vi "Vision 표지판 인식.vi"() -> ()   [LabVIEW 2016]
uses:
  <vilib>/vision/Classification.llb/IMAQ Classifier Nearest Neighbor options.ctl
  <vilib>/vision/NI_Vision_Development_Module.lvlib
  <vilib>/ptbypt/NI_PtbyPt.lvlib
panel:
  in  "Colors (Green)":u32[](array[colorbox])=[65280]
  in  "경로 설정":enum32{"주차", "유턴", "곡선", "동적"}(tab)
  in  "File Path (Particle Classification 1)":path=path "C:/Users/SeongHyeon/Desktop/[Github]_GPS Team/labview_program/작업중인 모든 Vi, dll파일 모음/전체프로그램/Sub Vi/Sensor/Vision Reference/주차.clf"
  in  "유턴File Path":path=path "C:/Users/SeongHyeon/Desktop/[Github]_GPS Team/labview_program/작업중인 모든 Vi, dll파일 모음/전체프로그램/Sub Vi/Sensor/Vision Reference/유턴2.clf"
  in  "곡선File Path 2":path=path "C:/Users/SeongHyeon/Desktop/[Github]_GPS Team/labview_program/작업중인 모든 Vi, dll파일 모음/전체프로그램/Sub Vi/Sensor/Vision Reference/곡선2.clf"
  in  "동적장애물File Path 4":path=path "C:/Users/SeongHyeon/Desktop/[Github]_GPS Team/labview_program/작업중인 모든 Vi, dll파일 모음/전체프로그램/Sub Vi/Sensor/Vision Reference/동적 장애물 Dark.clf"
  in  "Parameter 설정":enum32{"주차", "유턴", "곡선", "동적"}(tab)
  in  "주차 Paramaters":T2={"Preprocessing Options"={"Method"=-1, "Looking for"=1, "Threshold Range"={"Lower value"=0.0, "Upper value"=0.0}, "Threshold Limits"={"Lower value"=0.0, "Upper value"=0.0}, "Reject Border"=FALSE, "# of Erosions"=0, "Kernel Size"={"Lower value"=0, "Upper value"=0}, "Deviation Factor"=0.0}, "Nearest Neighbor Options"={"Method"=0, "Metric"=0, "k"=0}, "Particle Options"={"Scale Dependant"=FALSE, "Scale Factor"=0.0, "Symmetry Dependant"=FALSE, "Symmetry Factor"=0.0}} {"Preprocessing Options"."Deviation Factor" min=0.0; "Preprocessing Options"."Threshold Limits"."Upper value" format="%.2f"; "Preprocessing Options"."Threshold Limits"."Lower value" format="%.2f"; "Preprocessing Options"."Threshold Range"."Upper value" format="%.2f"; "Preprocessing Options"."Threshold Range"."Lower value" format="%.2f"; "Preprocessing Options"."# of Erosions" min=0; "Preprocessing Options"."Method" items=["Manual Threshold"=-1, "-"=-2, "Auto Threshold: Clustering"=0, "Auto Threshold: Entropy"=1, "Auto Threshold: Metric"=2, "Auto Threshold: Moments"=3, "Auto Threshold: Inter-class Variance"=4, "--"=-3, "Local Threshold: Niblack"=5, "Local Threshold: BG Correction"=6]; "Preprocessing Options"."Looking for" items=["Bright Objects", "Dark Objects"]; "Nearest Neighbor Options"."Method" items=["Nearest Neighbor", "K Nearest Neighbor", "Minimum Mean Distance"]; "Nearest Neighbor Options"."Metric" items=["Maximum", "Sum", "Euclidean"]; "Nearest Neighbor Options"."k" min=3}
  in  "유턴 Paramaters":T2={"Preprocessing Options"={"Method"=-1, "Looking for"=1, "Threshold Range"={"Lower value"=0.0, "Upper value"=0.0}, "Threshold Limits"={"Lower value"=0.0, "Upper value"=0.0}, "Reject Border"=FALSE, "# of Erosions"=0, "Kernel Size"={"Lower value"=0, "Upper value"=0}, "Deviation Factor"=0.0}, "Nearest Neighbor Options"={"Method"=0, "Metric"=0, "k"=0}, "Particle Options"={"Scale Dependant"=FALSE, "Scale Factor"=0.0, "Symmetry Dependant"=FALSE, "Symmetry Factor"=0.0}} {"Preprocessing Options"."Deviation Factor" min=0.0; "Preprocessing Options"."Threshold Limits"."Upper value" format="%.2f"; "Preprocessing Options"."Threshold Limits"."Lower value" format="%.2f"; "Preprocessing Options"."Threshold Range"."Upper value" format="%.2f"; "Preprocessing Options"."Threshold Range"."Lower value" format="%.2f"; "Preprocessing Options"."# of Erosions" min=0; "Preprocessing Options"."Method" items=["Manual Threshold"=-1, "-"=-2, "Auto Threshold: Clustering"=0, "Auto Threshold: Entropy"=1, "Auto Threshold: Metric"=2, "Auto Threshold: Moments"=3, "Auto Threshold: Inter-class Variance"=4, "--"=-3, "Local Threshold: Niblack"=5, "Local Threshold: BG Correction"=6]; "Preprocessing Options"."Looking for" items=["Bright Objects", "Dark Objects"]; "Nearest Neighbor Options"."Method" items=["Nearest Neighbor", "K Nearest Neighbor", "Minimum Mean Distance"]; "Nearest Neighbor Options"."Metric" items=["Maximum", "Sum", "Euclidean"]; "Nearest Neighbor Options"."k" min=3}
  in  "곡선 Paramaters":T2={"Preprocessing Options"={"Method"=-1, "Looking for"=1, "Threshold Range"={"Lower value"=0.0, "Upper value"=0.0}, "Threshold Limits"={"Lower value"=0.0, "Upper value"=0.0}, "Reject Border"=FALSE, "# of Erosions"=0, "Kernel Size"={"Lower value"=0, "Upper value"=0}, "Deviation Factor"=0.0}, "Nearest Neighbor Options"={"Method"=0, "Metric"=0, "k"=0}, "Particle Options"={"Scale Dependant"=FALSE, "Scale Factor"=0.0, "Symmetry Dependant"=FALSE, "Symmetry Factor"=0.0}} {"Preprocessing Options"."Deviation Factor" min=0.0; "Preprocessing Options"."Threshold Limits"."Upper value" format="%.2f"; "Preprocessing Options"."Threshold Limits"."Lower value" format="%.2f"; "Preprocessing Options"."Threshold Range"."Upper value" format="%.2f"; "Preprocessing Options"."Threshold Range"."Lower value" format="%.2f"; "Preprocessing Options"."# of Erosions" min=0; "Preprocessing Options"."Method" items=["Manual Threshold"=-1, "-"=-2, "Auto Threshold: Clustering"=0, "Auto Threshold: Entropy"=1, "Auto Threshold: Metric"=2, "Auto Threshold: Moments"=3, "Auto Threshold: Inter-class Variance"=4, "--"=-3, "Local Threshold: Niblack"=5, "Local Threshold: BG Correction"=6]; "Preprocessing Options"."Looking for" items=["Bright Objects", "Dark Objects"]; "Nearest Neighbor Options"."Method" items=["Nearest Neighbor", "K Nearest Neighbor", "Minimum Mean Distance"]; "Nearest Neighbor Options"."Metric" items=["Maximum", "Sum", "Euclidean"]; "Nearest Neighbor Options"."k" min=3}
  in  "동적 Paramaters":T2={"Preprocessing Options"={"Method"=-1, "Looking for"=1, "Threshold Range"={"Lower value"=0.0, "Upper value"=0.0}, "Threshold Limits"={"Lower value"=0.0, "Upper value"=0.0}, "Reject Border"=FALSE, "# of Erosions"=0, "Kernel Size"={"Lower value"=0, "Upper value"=0}, "Deviation Factor"=0.0}, "Nearest Neighbor Options"={"Method"=0, "Metric"=0, "k"=0}, "Particle Options"={"Scale Dependant"=FALSE, "Scale Factor"=0.0, "Symmetry Dependant"=FALSE, "Symmetry Factor"=0.0}} {"Preprocessing Options"."Deviation Factor" min=0.0; "Preprocessing Options"."Threshold Limits"."Upper value" format="%.2f"; "Preprocessing Options"."Threshold Limits"."Lower value" format="%.2f"; "Preprocessing Options"."Threshold Range"."Upper value" format="%.2f"; "Preprocessing Options"."Threshold Range"."Lower value" format="%.2f"; "Preprocessing Options"."# of Erosions" min=0; "Preprocessing Options"."Method" items=["Manual Threshold"=-1, "-"=-2, "Auto Threshold: Clustering"=0, "Auto Threshold: Entropy"=1, "Auto Threshold: Metric"=2, "Auto Threshold: Moments"=3, "Auto Threshold: Inter-class Variance"=4, "--"=-3, "Local Threshold: Niblack"=5, "Local Threshold: BG Correction"=6]; "Preprocessing Options"."Looking for" items=["Bright Objects", "Dark Objects"]; "Nearest Neighbor Options"."Method" items=["Nearest Neighbor", "K Nearest Neighbor", "Minimum Mean Distance"]; "Nearest Neighbor Options"."Metric" items=["Maximum", "Sum", "Euclidean"]; "Nearest Neighbor Options"."k" min=3}
  out "동적이냐":bool
  out "곡선이냐":bool
  out "횡단보도 거리":dbl[](array[numeric])
  out "유턴이냐":bool
  in  "ROI Descriptor (Particle Classification 1) 2":T3={"Global Rectangle"=[750, 250, 1250, 750], "Contours"=[{"ID"=enum."External", "Type"=3, "Coordinates"=[750, 399, 891, 593]}]} {"Contours"."Type" items=["No Selection", "Point", "Line", "Rectangle", "Oval", "Polygon", "Freehand Region", "Annulus", "Unused2", "Unused3", "Broken Line", "Freehand Line", "Rotated Rectangle"]}
  in  "Stop (F)":bool
  out "Image":T4(plugin-control)
  out "Identification Score":sgl
  out "주차냐":bool
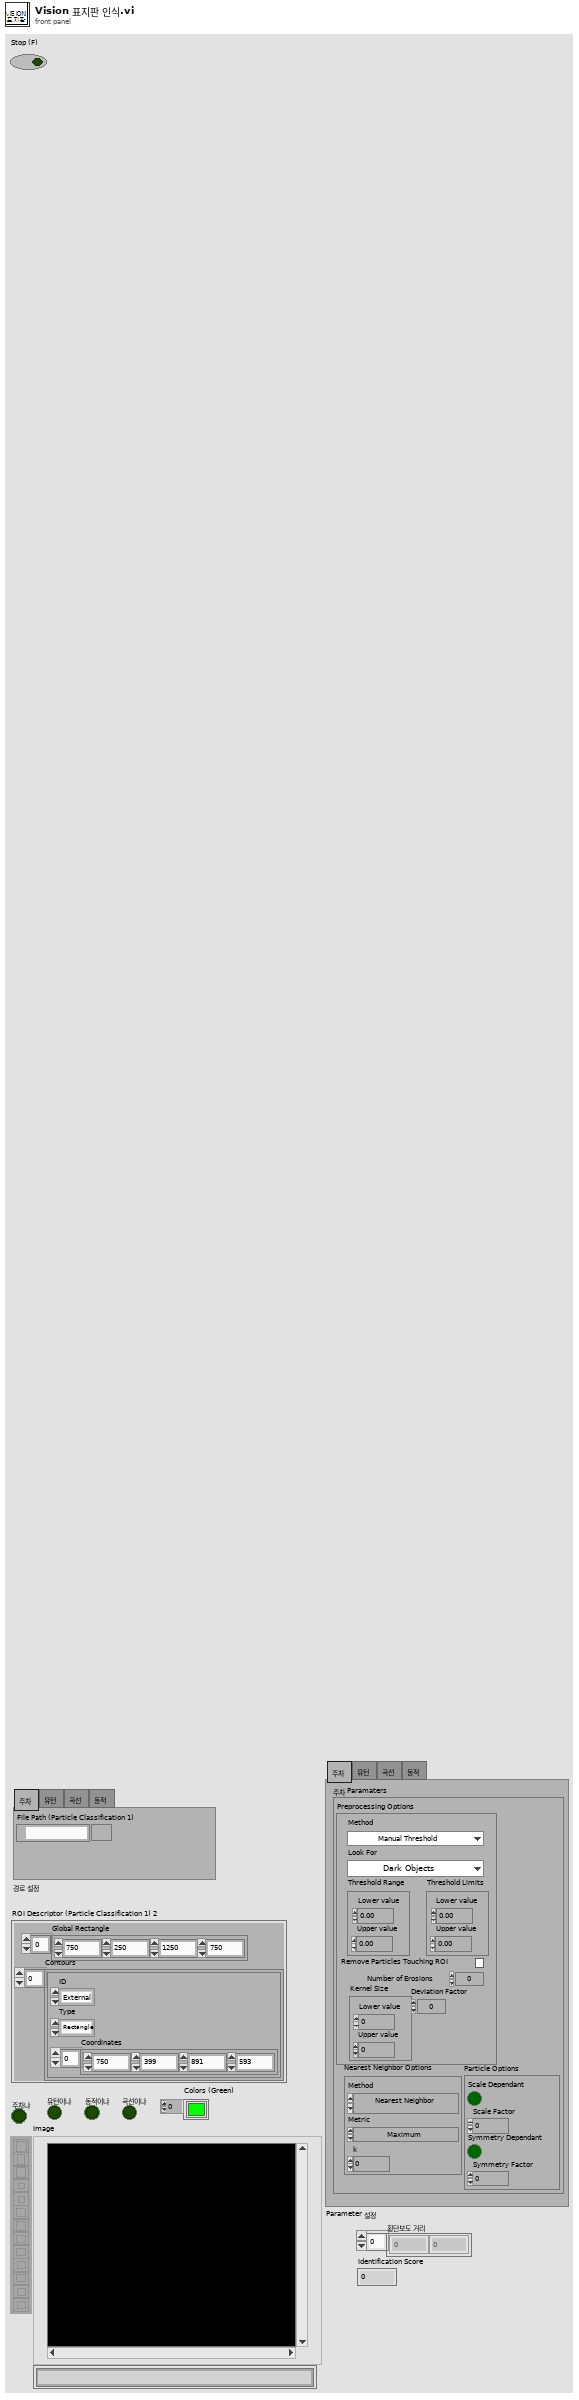
[diagram p1: front panel]
types:
  T1 = typedef "IMAQ Classifier Nearest Neighbor options.ctl" = cluster{"Method":i32, "Metric":i32, "k":i32}
  T2 = cluster{"Preprocessing Options":cluster{"Method":i32, "Looking for":i32, "Threshold Range":cluster{"Lower value":sgl, "Upper value":sgl}, "Threshold Limits":cluster{"Lower value":sgl, "Upper value":sgl}, "Reject Border":bool, "# of Erosions":i32, "Kernel Size":cluster{"Lower value":i32, "Upper value":i32}, "Deviation Factor":dbl}, "Nearest Neighbor Options":T1, "Particle Options":cluster{"Scale Dependant":bool, "Scale Factor":sgl, "Symmetry Dependant":bool, "Symmetry Factor":sgl}}
  T3 = cluster{"Global Rectangle":i32[], "Contours":cluster{"ID":enum32{"External", "Internal"}, "Type":u32, "Coordinates":i32[]}[]}
  T4 = typedef "IMAQ Image.ctl" = refnum<image>
  T5 = typedef "Image Type" = u32
  T6 = typedef "IMAQ Classifier Session.ctl" = refnum<k1>
  T7 = cluster{"Position":cluster{"x":sgl, "y":sgl}, "Angle":sgl, "Scale":sgl, "Score":sgl, "Bounding Box":cluster{"x":sgl, "y":sgl}[]}[]
  T8 = cluster{"Position":cluster{"x":sgl, "y":sgl}, "Angle":sgl, "Scale":sgl, "Score":sgl, "Bounding Box":cluster{"x":sgl, "y":sgl}[]}
  T9 = cluster{"Classification Score":sgl, "Identification Score":sgl}
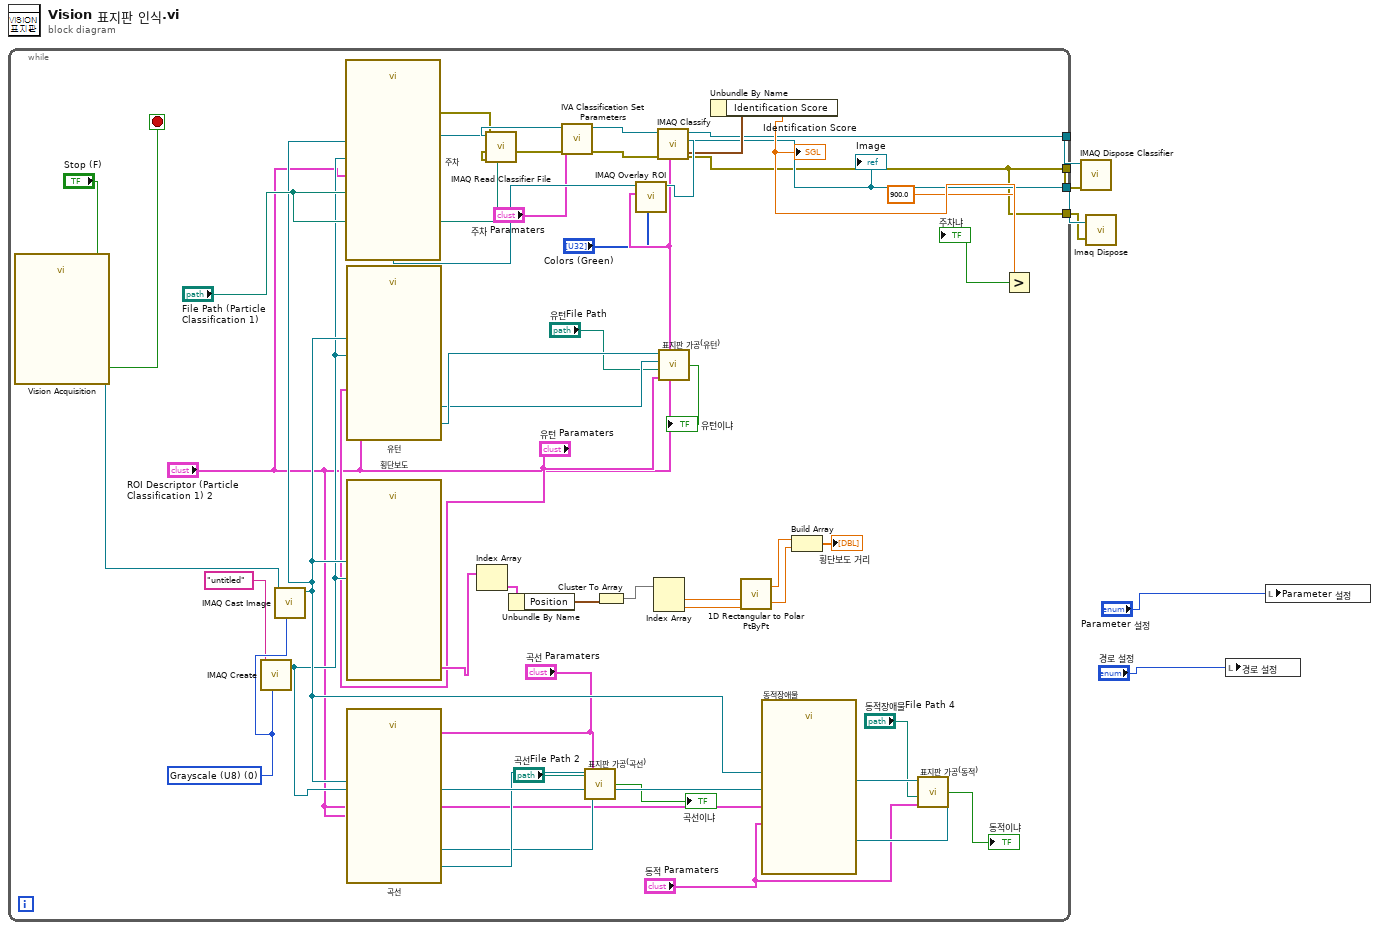
[diagram p0: block diagram]
diagram:
  n1 = while {
    tunnel: [w38] -> w6
    tunnel: [w36] -> w5
    tunnel: [w37] -> w4
    tunnel: [w36] -> w3
    stop <- w55 stop-if-true
    w53 = T5 0 items=["Grayscale (U8)", "Grayscale (I16)", "Grayscale (SGL)", "Complex (CSG)", "RGB (U32)", "HSL (U32)", "RGB (U64)", "Grayscale (U16)"] ("Image Type")
    n2 = call "Vision Acquisition"("Stop (F)"="Stop (F)") -> ("Image Out"=w54:T4, "Stopped"=w55:bool)  [unwired: 23 in, 2 out]
    n3 = call "IMAQ Create"("Image Name"="untitled", "Image Type"=w53) -> ("New Image"=w33:T4)  [unwired: 3 in, 1 out]
    n4 = call "IMAQ Cast Image"("Image Type"=w53, "Image Src"=w54) -> ("Image Dst Out"=w34:T4)  [unwired: 8 in, 1 out]
    n5 = call "주차"("Image In"=w34, "Image Dst"=w33, "ROI Descriptor (Particle Classification 1)"="ROI Descriptor (Particle Classification 1) 2", "File Path (Particle Classification 1)"="File Path (Particle Classification 1)") -> ("Image Out"=w42:T4, "Classifier Session (Particle Classification 1)"=w40:T6, "error out"=w39:errorcluster)  [unwired: 21 in]
    n6 = call "유턴"("Image In"=w34, "Image Dst"=w33, "ROI Descriptor (Particle Classification 1)"="ROI Descriptor (Particle Classification 1) 2", "Parameters (Particle Classification 1)"="유턴 Paramaters") -> ("Image Out"=w32:T4, "Classifier Session (Particle Classification 1)"=w31:T6)  [unwired: 21 in, 1 out]
    n7 = call "횡단보도"("Image In"=w34, "Image Dst"=w33) -> ("Calibrated Matches (Pattern Matching 1)"=w26:T7)  [unwired: 23 in, 2 out]
    n8 = call "곡선"("Image In"=w34, "ROI Descriptor (Particle Classification 1)"="ROI Descriptor (Particle Classification 1) 2", "Parameters (Particle Classification 1)"="곡선 Paramaters") -> ("Image Out"=w28:T4, "Classifier Session (Particle Classification 1)"=w17:T6)  [unwired: 22 in, 1 out]
    n9 = Index Array(array=w26) -> (element=w25:T8)  [unwired: 1 in]
    n10 = call "IMAQ Read Classifier File"("File Path"="File Path (Particle Classification 1)", "error in (no error)"=w39, "Classifier Session (optional)"=w40) -> ("error out"=w48:errorcluster, "Classifier Session"=w49:T6)  [unwired: 4 in, 3 out]
    n11 = Unbundle By Name(w25) -> ("Position"=w24:cluster{"x":sgl, "y":sgl})
    n12 = call <vilib>:"IVA Classification Set Parameters.vi"("error in"=w48, "Paramaters"="주차 Paramaters", "Classifier Session In"=w49) -> ("error out"=w47:errorcluster, "Classifier Session Out"=w43:T6)  [unwired: 7 out]
    n13 = call "표지판 가공(곡선).vi"("Paramaters"="곡선 Paramaters", "File Path"="곡선File Path 2", "Classifier Session (optional)"=w17, "Image 2"=w28) -> ("주차냐"=→"곡선이냐":bool)
    n14 = Cluster To Array(cluster=w24) -> (array=w23:sgl[])
    n15 = call "IMAQ Overlay ROI"("Colors (Green)"="Colors (Green)", "ROI Descriptor"="ROI Descriptor (Particle Classification 1) 2", "Image"=w42) -> ("Image Out"=w51:T4)  [unwired: 7 in, 1 out]
    n16 = Index Array(array=w23) -> (element #1=w22:sgl, element #2=w21:sgl)  [unwired: 2 in]
    n17 = call "IMAQ Classify"("ROI Descriptor"="ROI Descriptor (Particle Classification 1) 2", "error in (no error)"=w47, "Image"=w51, "Classifier Session"=w43) -> ("error out"=w36:errorcluster, "Image (dup)"=w37:T4, "Classifier Session (dup)"=w38:T6, "Scores"=w50:T9)  [unwired: 2 in, 2 out]
    "Image" <- w37
    n18 = call "표지판 가공(유턴).vi"("Paramaters"="유턴 Paramaters", "File Path"="유턴File Path", "Classifier Session (optional)"=w31, "Image 2"=w32) -> ("주차냐"=→"유턴이냐":bool)
    n19 = Unbundle By Name(w50) -> ("Identification Score"=w46:sgl)
    "Identification Score" <- w46
    n20 = call <vilib>:"1D Rectangular to Polar PtByPt.vi"("y"=w21, "x"=w22) -> ("phase"=w19:dbl, "magnitude"=w20:dbl)
    n21 = call "동적장애물"("Image In"=w34, "Image Dst"=w33, "ROI Descriptor (Particle Classification 1)"="ROI Descriptor (Particle Classification 1) 2", "Parameters (Particle Classification 1)"="동적 Paramaters") -> ("Image Out"=w15:T4, "Classifier Session (Particle Classification 1)"=w14:T6)  [unwired: 21 in, 1 out]
    n22 = Build Array(w20, w19) -> (→"횡단보도 거리":dbl[])
    n23 = call "표지판 가공(동적).vi"("Paramaters"="동적 Paramaters", "File Path"="동적장애물File Path 4", "Classifier Session (optional)"=w14, "Image 2"=w15) -> ("주차냐"=→"동적이냐":bool)
    n24 = Greater?(x=w46, y=sgl 900.0) -> (0:→"주차냐":bool)
  }
  n25 = call "IMAQ Dispose Classifier"("error in (no error)"=w5, "Classifier Session"=w6) -> ()  [unwired: 9 in, 1 out]
  n26 = call "Imaq Dispose"("Image"=w4, "error in (no error)"=w3) -> ()  [unwired: 4 in, 1 out]
  n27 = local write "경로 설정"("경로 설정") -> ()
  n28 = local write "Parameter 설정"("Parameter 설정") -> ()
